vi "event.create_programmatic.from_data_source.vi"(4 "Additional Information":T1, 5 "Duration (0s)":dbl, 6 "Properties and Labels":T2, 7 "Time Stamp (now: system time)":timestamp format="%<%x %.3X>T", 8 "error in":errorcluster, 9 "Name":string, 10 "Datasource RID":string, 11 "Nominal Client in":refnum<class "Nominal Client.lvclass">) -> (0 "error out":errorcluster, 3 "Nominal Client out":refnum<class "Nominal Client.lvclass">)   [LabVIEW 2020, in "Nominal Client.lvclass"]
doc: "Creates a timestamped event in Nominal associated with one or more assets, marking significant occurrences during test execution such as hardware state changes or sequence transitions. Events appear alongside telemetry data to enable correlation between test activities and system behavior during analysis."
uses:
  Nominal Client.lvclass
  asset/asset.lvclass
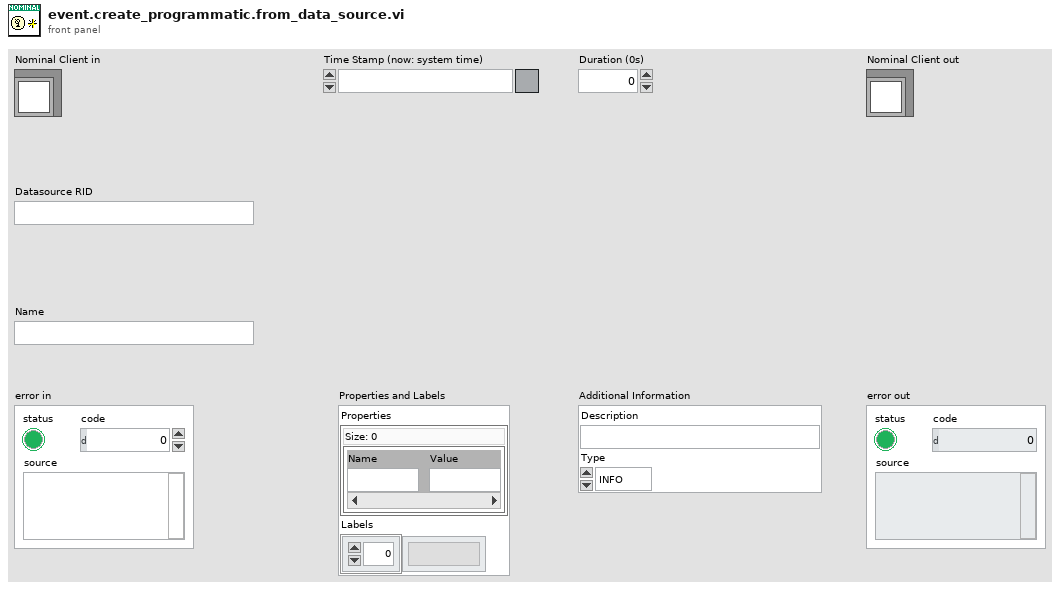
[diagram p1: front panel]
types:
  T1 = cluster{"Description":string, "Type":enum16{"INFO", "FLAG", "ERROR", "SUCCESS"}}
  T2 = cluster{"Properties":map{string, string}, "Labels":string[]}
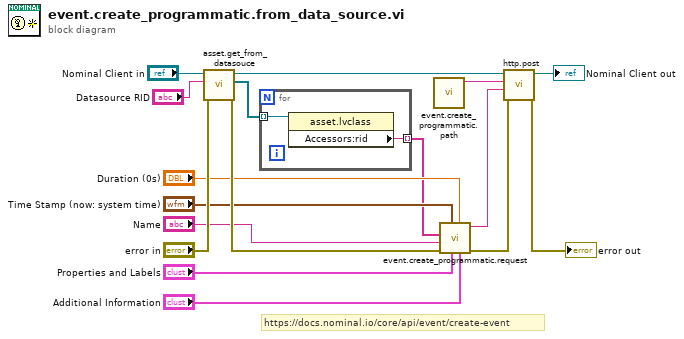
[diagram p0: block diagram]
diagram:
  # "https://docs.nominal.io/core/api/event/create-event"
  n1 = call "asset.get_from_datasouce.vi"("error in"="error in", "Datasource RID"="Datasource RID", "Nominal Client in"="Nominal Client in") -> ("error out"=w16:errorcluster, "Assets"=w4:refnum<class "asset.lvclass">[], "Nominal Client out"=w2:refnum<class "Nominal Client.lvclass">)  [unwired: 6 in]
  n2 = for {
    tunnel: w4 -> [w19] mode=indexing
    tunnel: [w18] -> w3 mode=indexing
    n3 = property class="asset.lvclass"(reference=w19) -> ("Accessors:rid"=w18:string)  [unwired: 1 in, 2 out]
  }
  n4 = call "event.create_programmatic.path.vi"() -> ("path"=w13:string)  [unwired: 11 in]
  n5 = call "event.create_programmatic.request.vi"("Additional Information"="Additional Information", "Duration (0s)"="Duration (0s)", "Properties and Labels"="Properties and Labels", "Time Stamp (now: system time)"="Time Stamp (now: system time)", "error in"=w16, "Name"="Name", "Asset RIDs"=w3) -> ("error out"=w8:errorcluster, "request"=w9:string)  [unwired: 3 in]
  n6 = call "http.post.vi"("error in"=w8, "Request body"=w9, "Path"=w13, "Nominal Client in"=w2) -> ("error out"=→"error out":errorcluster, "Nominal Client out"=→"Nominal Client out":refnum<class "Nominal Client.lvclass">)  [unwired: 4 in, 2 out]
